vi "FlexRIO GSE Bitfile Directory.vi"() -> (3 "Flexrio GSE Template Bitfiles Folder Path":path)   [LabVIEW 2025, in "I2C Bus Monitor UI.lvlib"]
uses:
  I2C Bus Monitor UI.lvlib
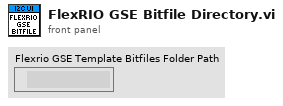
[diagram p1: front panel]
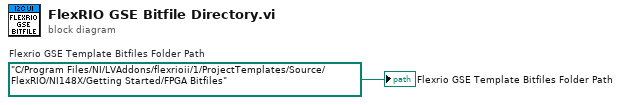
[diagram p0: block diagram]
diagram:
  w1 = path "C:/Program Files/NI/LVAddons/flexrioii/1/ProjectTemplates/Source/FlexRIO/NI148X/Getting Started/FPGA Bitfiles"  # Flexrio GSE Template Bitfiles Folder Path
  "Flexrio GSE Template Bitfiles Folder Path" <- w1
